vi "Init Setter.vi"(8 "error in (no error)":errorcluster, 9 "Setter Path":path, 10 "Class Type":refnum<class>, 11 "Binding in":refnum<class "Binding.lvclass">) -> (0 "error out":errorcluster, 3 "Binding out":refnum<class "Binding.lvclass">)   [LabVIEW 2020, in "PropertyBinder.lvlib" / "Binding.lvclass"]
uses:
  Binding.lvclass
  Setter Terminals.ctl
  Binding.lvclass/Binding.ctl
  PropertyBinder.lvlib
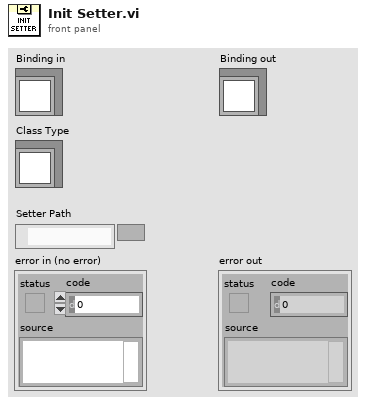
[diagram p1: front panel]
types:
  T1 = typedef "PropertyBinder.lvlib/Setter Terminals.ctl" = enum16{"Error out", "NC 1", "NC 2", "Class out", "NC 4", "NC 5", "NC 6", "NC 7", "Error in", "NC 9", "Value in", "Class in"}
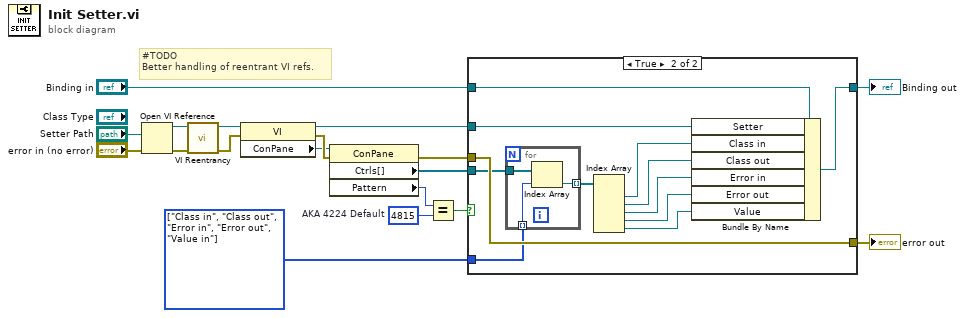
[diagram p0: block diagram]
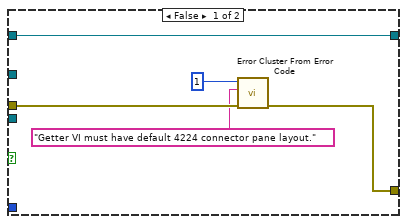
[diagram p2: hidden frame]
diagram:
  w11 = T1[] [enum."Class in", enum."Class out", enum."Error in", enum."Error out", enum."Value in"] items=["Error out", "NC 1", "NC 2", "Class out", "NC 4", "NC 5", "NC 6", "NC 7", "Error in", "NC 9", "Value in", "Class in"]
  w15 = u32 4815  # AKA 4224 Default
  # "#TODO\nBetter handling of reentrant VI refs."
  n1 = Open VI Reference(vi path="Setter Path", error in (no error)="error in (no error)") -> (vi reference=w1:refnum<vi>, error out=w2:errorcluster)  [unwired: 4 in]
  n2 = call "VI Reentrancy.vi"("error in (no error)"=w2, "VI in"=w1) -> ("error out"=w9:errorcluster, "VI"=w17:refnum<vi>)  [unwired: 7 in, 1 out]
  n3 = property class="VI"(reference=w17, error in=w9) -> (reference out=w10:refnum<vi>, error out=w18:errorcluster, "ConPane"=w14:refnum<vi>)
  n4 = property class="ConPane"(reference=w14, error in=w18) -> (error out=w8:errorcluster, "Ctrls[]"=w12:refnum<vi>[], "Pattern"=w16:u32)  [unwired: 1 out]
  n5 = Equal?(x=w16, y=w15) -> (x = y?=w13:bool)
  n6 = case shown="True" w13 {
    tunnel: w12 -> [_ w34]
    tunnel: w11 -> [_ w33]
    tunnel: w10 -> [_ w28]
    tunnel: "Binding in" -> [w23 w32]
    tunnel: [w23 w31] -> w6
    tunnel: w8 -> [w22 w35]
    tunnel: [w19 w35] -> w5
    frame False {
      n7 = call <vilib>:"Error Cluster From Error Code.vi"("error in (no error)"=w22, "error message (\"\")"="Getter VI must have default 4224 connector pane layout." ("error message (\"\")"), "error code (0)"=1) -> ("error out"=w19:errorcluster)  [unwired: 6 in]
    }
    frame True {
      n8 = for {
        tunnel: w34 -> [w38]
        tunnel: w33 -> [w37] mode=indexing
        tunnel: [w36] -> w30 mode=indexing
        n9 = Index Array(array=w38, index=w37) -> (element=w36:refnum<vi>)
      }
      n10 = Index Array(array=w30) -> (element #1=w29:refnum<vi>, element #2=w27:refnum<vi>, element #3=w26:refnum<vi>, element #4=w25:refnum<vi>, element #5=w24:refnum<vi>)  [unwired: 5 in]
      n11 = Bundle By Name(cluster=w32, "Setter"=w28, "Class in"=w29, "Class out"=w27, "Error in"=w26, "Error out"=w25, "Value"=w24) -> (w31:refnum<class "Binding.lvclass">)
    }
  }
  "error out" <- w5
  "Binding out" <- w6
